vi "send_packet.vi"(8 "error in (no error)":errorcluster, 10 "w5500_pck in":T1, 11 "TCP Network Connection in":refnum<k5>) -> (0 "error out":errorcluster, 3 "TCP Network Connection out":refnum<k5>)   [LabVIEW 2021]
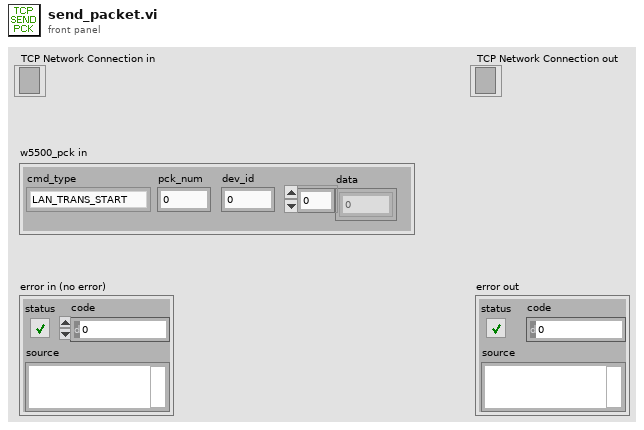
[diagram p1: front panel]
types:
  T1 = typedef "w5500_pck.ctl" = cluster{"cmd_type":T2, "pck_num":u32, "dev_id":u32, "data":u8[]}
  T2 = typedef "w5500_cmd.ctl" = enum32{"LAN_TRANS_START", "LAN_DATA_SZ", "LAN_CHUNK_SEND", "LAN_CHUNK_ACK", "LAN_DEVS_INFO", "LAN_DEVS_NUM", "LAN_DEVS_EXS", "LAN_DEVS_ACK", "LAN_CMD_ACK", "LAN_CMD_FIN", "LAN_SND_STAT", "LAN_REQ_STAT", "LAN_ANS_STAT", "LAN_ERR_STAT", "LAN_SETT_SET", "LAN_SETT_GET", "LAN_SETT_ACK", "LAN_SETT_ERR"}
  T3 = enum16{"big-endian, network order", "native, host order", "little-endian"}
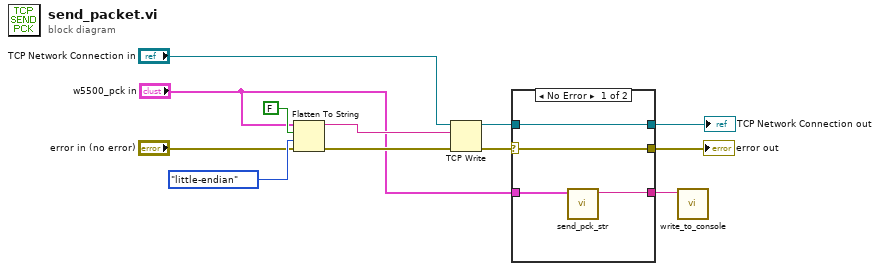
[diagram p0: block diagram]
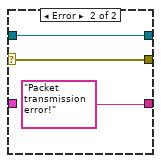
[diagram p2: hidden frame]
diagram:
  n1 = Flatten To String(anything="w5500_pck in", prepend array or string size? (T)=FALSE, byte order (0:big-endian, network order)=T3."little-endian", error in (no error)="error in (no error)") -> (data string=w2:string, error out=w10:errorcluster)  [unwired: 1 out]
  n2 = TCP Write(connection ID="TCP Network Connection in", data in=w2, error in (no error)=w10) -> (connection ID out=w5:refnum<k5>, error out=w6:errorcluster)  [unwired: 1 in, 1 out]
  n3 = case shown="No Error" w6 {
    selector: w6 -> [w16 w18]
    tunnel: [w16 w18] -> w3
    tunnel: [w14 "Packet transmission error!"] -> w7
    tunnel: w5 -> [w15 w17]
    tunnel: [w15 w17] -> w4
    tunnel: "w5500_pck in" -> [w13 _]
    frame No Error {
      n4 = call "send_pck_str.vi"("inp_pck"=w13) -> ("res_str"=w14:string)  [unwired: 10 in]
    }
    frame Error {
    }
  }
  "TCP Network Connection out" <- w4
  "error out" <- w3
  n5 = call "write_to_console.vi"("input_str"=w7) -> ()  [unwired: 9 in, 2 out]
